vi "Result_Test.vi"(8 "error in (no error)":errorcluster caption="entrée d'erreur (pas d'erreur)", 11 "Test (Default) en entrée":refnum<class "Test (Default).lvclass">) -> (0 "error out":errorcluster caption="sortie d'erreur", 3 "Test (Default) en sortie":refnum<class "Test (Default).lvclass">)   [LabVIEW 2020, in "Library Test.lvlib" / "Test (Default).lvclass"]
uses:
  Test (Default).lvclass
  Commun VI/TypeDef/Variable Printable.ctl
  Test (Default).lvclass/Test (Default).ctl
  Commun VI/Library Commun.lvlib
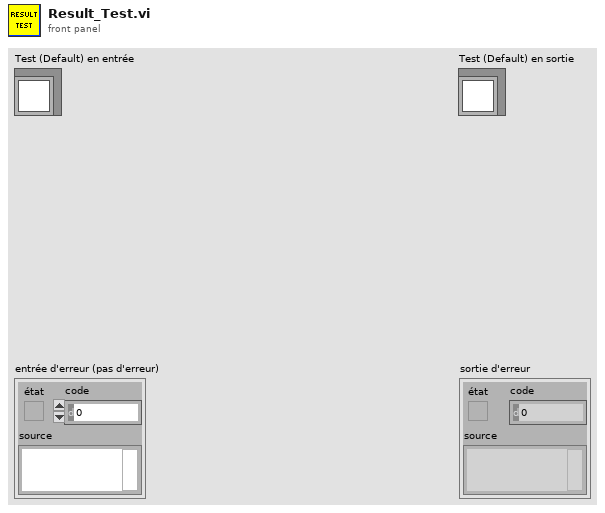
[diagram p1: front panel]
types:
  T1 = enum16{"Get Variable", "Get All Variables", "Set Variable", "Delete Variable", "Delete All Variable"}
  T2 = typedef "Variable Printable.ctl" = string
  T3 = typedef "Library Commun.lvlib/Commande Type Test.ctl" = enum16{"Function", "Test", "Calculation"}
  T4 = typedef "Library Commun.lvlib/Commande Data Test.ctl" = cluster{"Main Test":string, "Name Test":string, "StartOfTest":string, "Value":string, "Limit_Low":string, "Limit_High":string, "Result":bool, "Fatal_Test":bool, "NbRetry":dbl, "EndOfTest":string, "Error":string, "TypeValue":T5, "Type Test":T3}
  T5 = typedef "Library Commun.lvlib/Commande Value Type.ctl" = enum16{"None", "String", "Number", "Timestamp", "Boolean", "Array"}
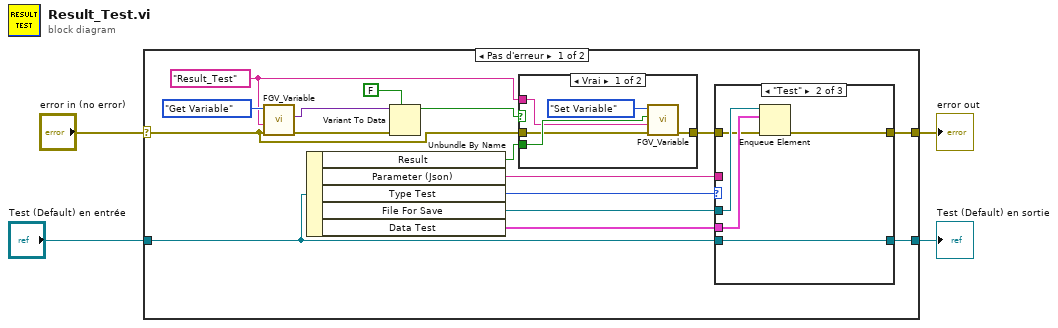
[diagram p0: block diagram]
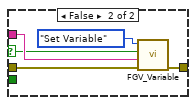
[diagram p2: hidden frame]
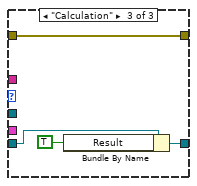
[diagram p4: hidden frame]
diagram:
  n1 = case shown="Pas d'erreur" "error in (no error)" {
    selector: "error in (no error)" -> [w5 w43]
    tunnel: [w19 w43] -> w3
    tunnel: [w20 w42] -> w1
    tunnel: "Test (Default) en entrée" -> [w18 w42]
    frame No Error {
      w8 = T2 "Result_Test" ("Variable")
      n2 = call "FGV_Variable.vi"("error in (no error)"=w5, "Variable"=w8, "Function"=T1."Get Variable") -> ("error out"=w12:errorcluster, "Data Out"=w11:variant)  [unwired: 6 in, 1 out]
      n3 = Unbundle By Name(w18) -> ("Result"=w9:bool, "Parameter (Json)"=w17:string, "Type Test"=w16:T3, "File For Save"=w15:refnum<queue>, "Data Test"=w14:T4)
      n4 = Variant To Data(error in=w12, type=FALSE, Variant=w11) -> (data=w7:bool)  [unwired: 1 out]
      n5 = case shown="Vrai" w7 {
        selector: w7 -> [_ w26]
        tunnel: w9 -> [w24 _]
        tunnel: [w23 w29] -> w6
        tunnel: w8 -> [w22 w28]
        tunnel: w5 -> [w21 w27]
        frame True {
          n6 = call "FGV_Variable.vi"("error in (no error)"=w21, "Variable"=w22, "Data In"=w24, "Function"=T1."Set Variable") -> ("error out"=w23:errorcluster)  [unwired: 5 in, 2 out]
        }
        frame False {
          n7 = call "FGV_Variable.vi"("error in (no error)"=w27, "Variable"=w28, "Data In"=w26, "Function"=T1."Set Variable") -> ("error out"=w29:errorcluster)  [unwired: 5 in, 2 out]
        }
      }
      n8 = case shown="\"Test\"" w16 {
        tunnel: [w31 w37 w41] -> w20
        tunnel: w18 -> [w31 w37 w39]
        tunnel: w17 -> [_ _ _]
        tunnel: w6 -> [w32 w34 w38]
        tunnel: [w32 w33 w38] -> w19
        tunnel: w15 -> [_ w36 _]
        tunnel: w14 -> [_ w35 _]
        frame "Function", Default {
        }
        frame "Test" {
          n9 = Enqueue Element(queue=w36, element=w35, error in (no error)=w34) -> (error out=w33:errorcluster)  [unwired: 1 in, 2 out]
        }
        frame "Calculation" {
          n10 = Bundle By Name(cluster=w39, "Result"=TRUE ("Data Test.Result")) -> (w41:refnum<class "Test (Default).lvclass">)
        }
      }
    }
    frame Error {
    }
  }
  "error out" <- w3
  "Test (Default) en sortie" <- w1
